vi "Autonomous Independent.vi"   [LabVIEW 2017] (continued)
                        frame #5 {
                          n2054 = global write "Robot Global Data.vi" "Current State"(TRUE ("Current State")) -> ()
                          n2055 = Wait (ms)(milliseconds to wait=u32 300) -> ()  [unwired: 1 out]
                        }
                      }
                    }
                    frame "L" {
                      n2056 = flat-sequence {
                        tunnel: w6977 -> [w6994]
                        tunnel: w6976 -> [w6993]
                        tunnel: [w6996] -> w6991
                        tunnel: [w6995] -> w6990
                        tunnel: w6991 -> [w7003]
                        tunnel: w6990 -> [w7002]
                        tunnel: [w7003] -> w6986
                        tunnel: [w7002] -> w6987
                        tunnel: [w7000] -> w6988
                        tunnel: [w6999] -> w6989
                        tunnel: w6974 -> [w6998]
                        tunnel: w6975 -> [w6997]
                        tunnel: w6989 -> [w7004]
                        tunnel: w6988 -> [w7005]
                        tunnel: w6987 -> [w7008]
                        tunnel: w6986 -> [w7009]
                        tunnel: [w7007] -> w6985
                        tunnel: [w7006] -> w6984
                        tunnel: [w7005] -> w6983
                        tunnel: [w7004] -> w6982
                        tunnel: w6985 -> [w7037]
                        tunnel: [w7037] -> w6981
                        tunnel: w6984 -> [w7036]
                        tunnel: [w7036] -> w6980
                        tunnel: w6983 -> [w7035]
                        tunnel: [w7033] -> w6979
                        tunnel: w6982 -> [w7034]
                        tunnel: [w7032] -> w6978
                        tunnel: w6981 -> [w7047]
                        tunnel: w6980 -> [w7046]
                        tunnel: w6979 -> [w7041]
                        tunnel: w6978 -> [w7039]
                        tunnel: [w7045] -> w6971
                        tunnel: [w7044] -> w6968
                        tunnel: [w7040] -> w6965
                        tunnel: [w7038] -> w6962
                        tunnel: w6961 -> [w7043]
                        tunnel: [w7052] -> w6972
                        tunnel: w6971 -> [w7052]
                        tunnel: [w7051] -> w6969
                        tunnel: w6968 -> [w7051]
                        tunnel: [w7050] -> w6966
                        tunnel: w6965 -> [w7050]
                        tunnel: [w7049] -> w6963
                        tunnel: w6962 -> [w7049]
                        tunnel: [w7065] -> w6973
                        tunnel: w6972 -> [w7065]
                        tunnel: [w7064] -> w6970
                        tunnel: w6969 -> [w7064]
                        tunnel: [w7061] -> w6967
                        tunnel: w6966 -> [w7063]
                        tunnel: [w7060] -> w6964
                        tunnel: w6963 -> [w7062]
                        tunnel: [w7055] -> w6960
                        tunnel: w6973 -> [w7079]
                        tunnel: w6970 -> [w7078]
                        tunnel: w6967 -> [w7077]
                        tunnel: w6964 -> [w7076]
                        tunnel: w6960 -> [w7074]
                        frame #0 {
                          n2057 = call "PID turning.vi"("Angle"=170.0, "GyroDevRef"=w6993, "RobotDriveDevRef"=w6994) -> ("GyroDevRef 2"=w6995:T8, "RobotDriveDevRef 2"=w6996:T1)  [unwired: 7 in]
                        }
                        frame #1 {
                          n2058 = call <vilib>:"WPI_EncoderReset.vi"("EncoderDevRef"=w6998) -> ("EncoderDevRef"=w6999:T11)  [unwired: 9 in, 1 out]
                          n2059 = Wait (ms)(milliseconds to wait=u32 10) -> ()  [unwired: 1 out]
                          n2060 = call <vilib>:"WPI_EncoderReset.vi"("EncoderDevRef"=w6997) -> ("EncoderDevRef"=w7000:T11)  [unwired: 9 in, 1 out]
                        }
                        frame #2 {
                          n2061 = global read "Robot Global Data.vi" "Axes"() -> (w7016:dbl[])
                          n2062 = Wait (ms)(milliseconds to wait=u32 400) -> ()  [unwired: 1 out]
                          n2063 = Array To Cluster(array=w7016) -> (cluster=w7017:T15)
                          n2064 = global read "Robot Global Data.vi" "PIXY Output"() -> (w7010:T16)
                          n2065 = Bundle By Name(cluster=w7017, "Axes[1]"=1.0) -> (w7018:T15)
                          n2066 = Unbundle By Name(w7010) -> ("SIGNATURE NUMBER"=w7013:u16)
                          n2067 = global read "Robot Global Data.vi" "Cube Signature"() -> (w7012:dbl)
                          n2068 = Equal?(x=w7013, y=w7012) -> (x = y?=w7011:bool)
                          n2069 = Cluster To Array(cluster=w7018) -> (array=w7019:dbl[])
                          n2070 = global write "Robot Global Data.vi" "Axes"(w7019) -> ()
                          n2071 = case shown="True" w7011 {
                            tunnel: [w7026 w7029] -> w7006
                            tunnel: [w7027 w7028] -> w7007
                            tunnel: w7009 -> [w7021 w7028]
                            tunnel: w7008 -> [w7020 w7029]
                            frame True {
                              n2072 = call <vilib>:"WPI_GyroGetAngle.vi"("GyroDevRef"=w7020) -> ("Angle"=w7025:dbl, "GyroDevRef"=w7026:T8)  [unwired: 6 in, 3 out]
                              n2073 = In Range and Coerce(upper limit=170.0, x=w7025, lower limit=155.0) -> (coerced(x)=w7024:dbl)  [unwired: 1 out]
                              n2074 = global write "Robot Global Data.vi" "Tracked Angle"(w7024) -> ()
                              n2075 = call "PID vision.vi"("RobotDriveDevRef in"=w7021) -> ("RobotDriveDevRef out"=w7027:T1)  [unwired: 9 in, 1 out]
                            }
                            frame False {
                              n2076 = global write "Robot Global Data.vi" "Tracked Angle"(170.0) -> ()
                            }
                          }
                        }
                        frame #3 {
                          n2077 = call <vilib>:"WPI_EncoderReset.vi"("EncoderDevRef"=w7034) -> ("EncoderDevRef"=w7032:T11)  [unwired: 9 in, 1 out]
                          n2078 = Wait (ms)(milliseconds to wait=u32 10) -> ()  [unwired: 1 out]
                          n2079 = call <vilib>:"WPI_EncoderReset.vi"("EncoderDevRef"=w7035) -> ("EncoderDevRef"=w7033:T11)  [unwired: 9 in, 1 out]
                        }
                        frame #4 {
                          n2080 = global read "Robot Global Data.vi" "Tracked Angle"() -> (w7048:dbl)
                          n2081 = call "PID with Infrared.vi"("RobotDriveDevRef"=w7047, "Angle"=w7048, "Encoder Limit"=60.0, "GyroDevRef"=w7046, "Left Encoder"=w7041, "Right Encoder"=w7039, "DigitalInputDevRef"=w7043) -> ("RobotDriveDevRef 2"=w7045:T1, "GyroDevRef 2"=w7044:T8, "Left Encoder 2"=w7040:T11, "Right Encoder 2"=w7038:T11)  [unwired: 4 in, 1 out]
                        }
                        frame #5 {
                          n2082 = global write "Robot Global Data.vi" "Current State"(TRUE ("Current State")) -> ()
                          n2083 = Wait (ms)(milliseconds to wait=u32 500) -> ()  [unwired: 1 out]
                        }
                        frame #6 {
                          n2084 = global read "Robot Global Data.vi" "Axes"() -> (w7071:dbl[])
                          n2085 = global write "Robot Global Data.vi" "Lift_Position"(2.0) -> ()
                          n2086 = Wait (ms)(milliseconds to wait=u32 400) -> ()  [unwired: 1 out]
                          n2087 = Array To Cluster(array=w7071) -> (cluster=w7070:T15)
                          n2088 = Bundle By Name(cluster=w7070, "Axes[1]"=-1.0) -> (w7069:T15)
                          n2089 = call <vilib>:"WPI_EncoderGet.vi"("EncoderDevRef"=w7063) -> ("Distance"=w7059:dbl, "EncoderDevRef"=w7061:T11)  [unwired: 5 in, 4 out]
                          n2090 = call <vilib>:"WPI_EncoderGet.vi"("EncoderDevRef"=w7062) -> ("Distance"=w7058:dbl, "EncoderDevRef"=w7060:T11)  [unwired: 5 in, 4 out]
                          n2091 = Add(x=w7059, y=w7058) -> (x+y=w7057:dbl)
                          n2092 = Cluster To Array(cluster=w7069) -> (array=w7068:dbl[])
                          n2093 = global write "Robot Global Data.vi" "Axes"(w7068) -> ()
                          n2094 = Divide(x=w7057, y=2.0) -> (x/y=w7055:dbl)
                        }
                        frame #7 {
                          n2095 = Add(x=w7074, y=15.0 ("Distance")) -> (x+y=w7073:dbl)
                          n2096 = global read "Robot Global Data.vi" "Tracked Angle"() -> (w7080:dbl)
                          n2097 = call "PID Distance.vi"("Distance"=w7073, "Angle"=w7080, "RightEncoder"=w7076, "LeftEncoder"=w7077, "GyroDevRef"=w7078, "RobotDriveDevRef"=w7079) -> ()  [unwired: 2 in, 4 out]
                        }
                        frame #8 {
                          n2098 = global read "Robot Global Data.vi" "Axes"() -> (w7086:dbl[])
                          n2099 = Wait (ms)(milliseconds to wait=u32 200) -> ()  [unwired: 1 out]
                          n2100 = Array To Cluster(array=w7086) -> (cluster=w7085:T15)
                          n2101 = Bundle By Name(cluster=w7085, "Axes[1]"=0.5) -> (w7084:T15)
                          n2102 = Cluster To Array(cluster=w7084) -> (array=w7083:dbl[])
                          n2103 = global write "Robot Global Data.vi" "Axes"(w7083) -> ()
                        }
                        frame #9 {
                          n2104 = global write "Robot Global Data.vi" "Current State"(FALSE ("Current State")) -> ()
                        }
                      }
                    }
                    frame Default {
                    }
                  }
                }
              }
            }
            frame "R" {
              n2105 = flat-sequence {
                tunnel: [w7154] -> w7142
                tunnel: [w7153] -> w7143
                tunnel: [w7151] -> w7144
                tunnel: [w7152] -> w7145
                tunnel: w7101 -> [w7150]
                tunnel: w7100 -> [w7149]
                tunnel: w7099 -> [w7148]
                tunnel: w7098 -> [w7147]
                tunnel: [w7174] -> w7141
                tunnel: w7145 -> [w7170]
                tunnel: w7144 -> [w7171]
                tunnel: w7143 -> [w7173]
                tunnel: w7142 -> [w7175]
                tunnel: [w7172] -> w7140
                tunnel: [w7171] -> w7139
                tunnel: [w7170] -> w7138
                tunnel: w7141 -> [w7185]
                tunnel: [w7185] -> w7137
                tunnel: w7140 -> [w7184]
                tunnel: [w7184] -> w7136
                tunnel: [w7183] -> w7135
                tunnel: [w7182] -> w7134
                tunnel: w7139 -> [w7180]
                tunnel: w7138 -> [w7179]
                tunnel: w7137 -> [w7191]
                tunnel: [w7189] -> w7133
                tunnel: w7136 -> [w7190]
                tunnel: [w7188] -> w7132
                tunnel: w7135 -> [w7193]
                tunnel: w7134 -> [w7192]
                tunnel: [w7187] -> w7131
                tunnel: [w7186] -> w7130
                tunnel: w7133 -> [w7200]
                tunnel: [w7199] -> w7129
                tunnel: [w7198] -> w7128
                tunnel: w7132 -> [w7198]
                tunnel: [w7197] -> w7127
                tunnel: w7131 -> [w7197]
                tunnel: [w7196] -> w7126
                tunnel: w7130 -> [w7196]
                tunnel: [w7211] -> w7125
                tunnel: w7129 -> [w7211]
                tunnel: [w7210] -> w7124
                tunnel: w7128 -> [w7210]
                tunnel: [w7209] -> w7123
                tunnel: w7127 -> [w7209]
                tunnel: [w7208] -> w7122
                tunnel: w7126 -> [w7208]
                tunnel: w7125 -> [w7216]
                tunnel: w7124 -> [w7217]
                tunnel: [w7217] -> w7121
                tunnel: [w7216] -> w7120
                tunnel: [w7215] -> w7119
                tunnel: w7123 -> [w7215]
                tunnel: [w7214] -> w7118
                tunnel: w7122 -> [w7214]
                tunnel: [w7230] -> w7117
                tunnel: w7121 -> [w7232]
                tunnel: w7120 -> [w7231]
                tunnel: w7119 -> [w7227]
                tunnel: w7118 -> [w7226]
                tunnel: [w7225] -> w7116
                tunnel: [w7224] -> w7115
                tunnel: [w7223] -> w7114
                tunnel: w7117 -> [w7239]
                tunnel: w7116 -> [w7238]
                tunnel: [w7237] -> w7096
                tunnel: w7115 -> [w7237]
                tunnel: [w7236] -> w7094
                tunnel: w7114 -> [w7236]
                tunnel: [w7235] -> w7092
                tunnel: [w7234] -> w7090
                tunnel: w7096 -> [w7248]
                tunnel: [w7245] -> w7095
                tunnel: w7094 -> [w7247]
                tunnel: [w7244] -> w7093
                tunnel: w7092 -> [w7249]
                tunnel: [w7246] -> w7091
                tunnel: w7090 -> [w7243]
                tunnel: [w7242] -> w7088
                tunnel: w7095 -> [w7274]
                tunnel: w7093 -> [w7273]
                tunnel: [w7271] -> w7113
                tunnel: w7091 -> [w7271]
                tunnel: [w7268] -> w7112
                tunnel: [w7270] -> w7111
                tunnel: [w7269] -> w7110
                tunnel: w7088 -> [w7268]
                tunnel: w7113 -> [w7284]
                tunnel: w7112 -> [w7282]
                tunnel: w7111 -> [w7278]
                tunnel: w7110 -> [w7276]
                tunnel: [w7283] -> w7109
                tunnel: [w7281] -> w7108
                tunnel: [w7277] -> w7107
                tunnel: [w7275] -> w7106
                tunnel: w7089 -> [w7280]
                tunnel: [w7295] -> w7105
                tunnel: [w7292] -> w7104
                tunnel: [w7294] -> w7103
                tunnel: [w7293] -> w7102
                tunnel: w7106 -> [w7292]
                tunnel: w7107 -> [w7293]
                tunnel: w7108 -> [w7294]
                tunnel: w7109 -> [w7295]
                tunnel: w7105 -> [w7302]
                tunnel: w7104 -> [w7301]
                tunnel: w7103 -> [w7300]
                tunnel: w7102 -> [w7299]
                tunnel: w7097 -> [w7298]
                frame #0 {
                  n2106 = while {
                    tunnel: [w7159] -> w7146
                    stop <- w7158 stop-if-true
                    w7162 = 100.0 ("y")
                    w7165 = 20.0 ("y")
                    n2107 = global read "Robot Global Data.vi" "Distance 2"() -> (w7160:dbl)
                    n2108 = global read "Robot Global Data.vi" "Distance"() -> (w7161:dbl)
                    n2109 = Greater?(x=w7161, y=w7165) -> (0:w7167:bool)
                    n2110 = Greater?(x=w7160, y=w7165) -> (0:w7166:bool)
                    n2111 = Greater?(x=w7161, y=w7162) -> (0:w7164:bool)
                    n2112 = Greater?(x=w7160, y=w7162) -> (0:w7163:bool)
                    n2113 = Or(x=w7167, y=w7166) -> (x .or. y?=w7157:bool)
                    n2114 = Or(x=w7164, y=w7163) -> (x .or. y?=w7158:bool)
                    n2115 = global write "Robot Global Data.vi" "Raise_Mast"(w7157) -> ()
                    n2116 = case shown="True" w7158 {
                      tunnel: [0.0 2.0] -> w7159
                      frame False {
                      }
                      frame True {
                      }
                    }
                  }
                  n2117 = call "PID Distance.vi"("Distance"=295.0, "Angle"=2.0, "RightEncoder"=w7147, "LeftEncoder"=w7148, "GyroDevRef"=w7149, "RobotDriveDevRef"=w7150) -> ("RightEncoder 2"=w7151:T11, "LeftEncoder 2"=w7152:T11, "GyroDevRef 2"=w7153:T8, "RobotDriveDevRef 2"=w7154:T1)  [unwired: 2 in]
                  n2118 = global write "Robot Global Data.vi" "Lift_Position"(w7146) -> ()
                }
                frame #1 {
                  n2119 = call "PID turning.vi"("Angle"=-90.0, "GyroDevRef"=w7173, "RobotDriveDevRef"=w7175) -> ("GyroDevRef 2"=w7172:T8, "RobotDriveDevRef 2"=w7174:T1)  [unwired: 7 in]
                  n2120 = global write "Robot Global Data.vi" "Lift_Position"(3.0) -> ()
                  n2121 = global write "Robot Global Data.vi" "Raise_Mast"(TRUE ("Current State")) -> ()
                }
                frame #2 {
                  n2122 = call <vilib>:"WPI_EncoderReset.vi"("EncoderDevRef"=w7179) -> ("EncoderDevRef"=w7182:T11)  [unwired: 9 in, 1 out]
                  n2123 = Wait (ms)(milliseconds to wait=u32 100) -> ()  [unwired: 1 out]
                  n2124 = call <vilib>:"WPI_EncoderReset.vi"("EncoderDevRef"=w7180) -> ("EncoderDevRef"=w7183:T11)  [unwired: 9 in, 1 out]
                }
                frame #3 {
                  n2125 = call "PID Distance.vi"("Distance"=25.0, "Angle"=-90.0, "RightEncoder"=w7193, "LeftEncoder"=w7192, "GyroDevRef"=w7190, "RobotDriveDevRef"=w7191) -> ("RightEncoder 2"=w7186:T11, "LeftEncoder 2"=w7187:T11, "GyroDevRef 2"=w7188:T8, "RobotDriveDevRef 2"=w7189:T1)  [unwired: 2 in]
                }
                frame #4 {
                  w7201 = 0.0 ("Left axis value")
                  n2126 = global read "Robot Global Data.vi" "Axes"() -> (w7204:dbl[])
                  n2127 = Wait (ms)(milliseconds to wait=u32 500) -> ()  [unwired: 1 out]
                  n2128 = Array To Cluster(array=w7204) -> (cluster=w7203:T15)
                  n2129 = Bundle By Name(cluster=w7203, "Axes[1]"=0.25) -> (w7206:T15)
                  n2130 = Cluster To Array(cluster=w7206) -> (array=w7205:dbl[])
                  n2131 = call <vilib>:"WPI_RobotDriveTankDrive.vi"("Right axis value"=w7201, "Left axis value"=w7201, "RobotDriveDevRef"=w7200) -> ("RobotDriveDevRef"=w7199:T1)  [unwired: 6 in, 2 out]
                  n2132 = global write "Robot Global Data.vi" "Axes"(w7205) -> ()
                }
                frame #5 {
                  n2133 = global write "Robot Global Data.vi" "Current State"(FALSE ("Current State")) -> ()
                  n2134 = Wait (ms)(milliseconds to wait=u32 400) -> ()  [unwired: 1 out]
                }
                frame #6 {
                  n2135 = global read "Robot Global Data.vi" "Axes"() -> (w7219:dbl[])
                  n2136 = Array To Cluster(array=w7219) -> (cluster=w7218:T15)
                  n2137 = Bundle By Name(cluster=w7218, "Axes[1]"=-1.0) -> (w7221:T15)
                  n2138 = Cluster To Array(cluster=w7221) -> (array=w7220:dbl[])
                  n2139 = global write "Robot Global Data.vi" "Axes"(w7220) -> ()
                }
                frame #7 {
                  # "7 for A bot"
                  n2140 = call "PID Distance.vi"("Distance"=7.0, "Angle"=-90.0, "RightEncoder"=w7226, "LeftEncoder"=w7227, "GyroDevRef"=w7232, "RobotDriveDevRef"=w7231) -> ("RightEncoder 2"=w7223:T11, "LeftEncoder 2"=w7224:T11, "GyroDevRef 2"=w7225:T8, "RobotDriveDevRef 2"=w7230:T1)  [unwired: 2 in]
                }
                frame #8 {
                  n2141 = global write "Robot Global Data.vi" "Lift_Position"(1.0) -> ()
                  n2142 = call "PID turning.vi"("Angle"=-170.0, "GyroDevRef"=w7238, "RobotDriveDevRef"=w7239) -> ("GyroDevRef 2"=w7234:T8, "RobotDriveDevRef 2"=w7235:T1)  [unwired: 7 in]
                }
                frame #9 {
                  n2143 = global read "Robot Global Data.vi" "PIXY Output"() -> (w7252:T16)
                  n2144 = Unbundle By Name(w7252) -> ("SIGNATURE NUMBER"=w7251:u16)
                  n2145 = global read "Robot Global Data.vi" "Cube Signature"() -> (w7241:dbl)
                  n2146 = Equal?(x=w7251, y=w7241) -> (x = y?=w7250:bool)
                  n2147 = case shown="True" w7250 {
                    tunnel: [w7260 w7264] -> w7244
                    tunnel: [w7259 w7265] -> w7245
                    tunnel: [w7261 w7266] -> w7246
                    tunnel: w7248 -> [w7259 w7265]
                    tunnel: w7247 -> [w7260 w7264]
                    tunnel: w7249 -> [w7262 w7266]
                    tunnel: w7243 -> [w7254 w7263]
                    tunnel: [w7253 w7263] -> w7242
                    frame True {
                      # "-150_-170"
                      n2148 = call <vilib>:"WPI_GyroGetAngle.vi"("GyroDevRef"=w7254) -> ("Angle"=w7257:dbl, "GyroDevRef"=w7253:T8)  [unwired: 6 in, 3 out]
                      n2149 = In Range and Coerce(upper limit=-150.0, x=w7257, lower limit=-170.0) -> (coerced(x)=w7258:dbl)  [unwired: 1 out]
                      n2150 = global write "Robot Global Data.vi" "Tracked Angle"(w7258) -> ()
                      n2151 = call "PID vision.vi"("RobotDriveDevRef in"=w7262) -> ("RobotDriveDevRef out"=w7261:T1)  [unwired: 9 in, 1 out]
                    }
                    frame False {
                      n2152 = global write "Robot Global Data.vi" "Tracked Angle"(-165.0) -> ()
                    }
                  }
                }
                frame #10 {
                  n2153 = call <vilib>:"WPI_EncoderReset.vi"("EncoderDevRef"=w7274) -> ("EncoderDevRef"=w7270:T11)  [unwired: 9 in, 1 out]
                  n2154 = Wait (ms)(milliseconds to wait=u32 10) -> ()  [unwired: 1 out]
                  n2155 = call <vilib>:"WPI_EncoderReset.vi"("EncoderDevRef"=w7273) -> ("EncoderDevRef"=w7269:T11)  [unwired: 9 in, 1 out]
                }
                frame #11 {
                  n2156 = global write "Robot Global Data.vi" "Lift_Position"(0.0) -> ()
                  n2157 = global read "Robot Global Data.vi" "Axes"() -> (w7289:dbl[])
                  n2158 = Array To Cluster(array=w7289) -> (cluster=w7288:T15)
                  n2159 = global read "Robot Global Data.vi" "Tracked Angle"() -> (w7285:dbl)
                  n2160 = Bundle By Name(cluster=w7288, "Axes[1]"=1.0) -> (w7291:T15)
                  n2161 = call "PID with Infrared.vi"("RobotDriveDevRef"=w7284, "Angle"=w7285, "Encoder Limit"=120.0, "GyroDevRef"=w7282, "Left Encoder"=w7278, "Right Encoder"=w7276, "DigitalInputDevRef"=w7280) -> ("RobotDriveDevRef 2"=w7283:T1, "GyroDevRef 2"=w7281:T8, "Left Encoder 2"=w7277:T11, "Right Encoder 2"=w7275:T11)  [unwired: 4 in, 1 out]
                  n2162 = Cluster To Array(cluster=w7291) -> (array=w7290:dbl[])
                  n2163 = global write "Robot Global Data.vi" "Axes"(w7290) -> ()
                }
                frame #12 {
                  n2164 = global write "Robot Global Data.vi" "Current State"(TRUE ("Current State")) -> ()
                  n2165 = Wait (ms)(milliseconds to wait=u32 750) -> ()  [unwired: 1 out]
                }
                frame #13 {
                  n2166 = case shown="\"L\"" w7298 {
                    tunnel: w7302 -> [w7309 w7373 _]
                    tunnel: w7301 -> [w7306 w7372 _]
                    tunnel: w7300 -> [w7308 w7371 _]
                    tunnel: w7299 -> [w7307 w7370 _]
                    frame "R" {
                      n2167 = flat-sequence {
                        tunnel: w7307 -> [w7318]
                        tunnel: w7306 -> [w7317]
                        tunnel: [w7316] -> w7305
                        tunnel: [w7315] -> w7304
                        tunnel: [w7310] -> w7303
                        tunnel: w7309 -> [w7333]
                        tunnel: w7308 -> [w7332]
                        tunnel: w7305 -> [w7330]
                        tunnel: w7304 -> [w7329]
                        tunnel: w7303 -> [w7326]
                        frame #0 {
                          n2168 = global read "Robot Global Data.vi" "Axes"() -> (w7323:dbl[])
                          n2169 = global write "Robot Global Data.vi" "Lift_Position"(2.0) -> ()
                          n2170 = Wait (ms)(milliseconds to wait=u32 250) -> ()  [unwired: 1 out]
                          n2171 = Array To Cluster(array=w7323) -> (cluster=w7322:T15)
                          n2172 = Bundle By Name(cluster=w7322, "Axes[1]"=-1.0) -> (w7325:T15)
                          n2173 = call <vilib>:"WPI_EncoderGet.vi"("EncoderDevRef"=w7318) -> ("Distance"=w7314:dbl, "EncoderDevRef"=w7316:T11)  [unwired: 5 in, 4 out]
                          n2174 = call <vilib>:"WPI_EncoderGet.vi"("EncoderDevRef"=w7317) -> ("Distance"=w7313:dbl, "EncoderDevRef"=w7315:T11)  [unwired: 5 in, 4 out]
                          n2175 = Add(x=w7314, y=w7313) -> (x+y=w7312:dbl)
                          n2176 = Cluster To Array(cluster=w7325) -> (array=w7324:dbl[])
                          n2177 = global write "Robot Global Data.vi" "Axes"(w7324) -> ()
                          n2178 = Divide(x=w7312, y=2.0) -> (x/y=w7310:dbl)
                        }
                        frame #1 {
                          n2179 = Add(x=w7326, y=15.0 ("Distance")) -> (x+y=w7327:dbl)
                          n2180 = global read "Robot Global Data.vi" "Tracked Angle"() -> (w7331:dbl)
                          n2181 = call "PID Distance.vi"("Distance"=w7327, "Angle"=w7331, "RightEncoder"=w7329, "LeftEncoder"=w7330, "GyroDevRef"=w7332, "RobotDriveDevRef"=w7333) -> ()  [unwired: 2 in, 4 out]
                        }
                        frame #2 {
                          n2182 = global read "Robot Global Data.vi" "Axes"() -> (w7337:dbl[])
                          n2183 = Wait (ms)(milliseconds to wait=u32 200) -> ()  [unwired: 1 out]
                          n2184 = Array To Cluster(array=w7337) -> (cluster=w7336:T15)
                          n2185 = Bundle By Name(cluster=w7336, "Axes[1]"=0.5) -> (w7339:T15)
                          n2186 = Cluster To Array(cluster=w7339) -> (array=w7338:dbl[])
                          n2187 = global write "Robot Global Data.vi" "Axes"(w7338) -> ()
                        }
                        frame #3 {
                          n2188 = global write "Robot Global Data.vi" "Current State"(FALSE ("Current State")) -> ()
                          n2189 = Wait (ms)(milliseconds to wait=u32 500) -> ()  [unwired: 1 out]
                        }
                      }
                    }
                    frame "L" {
                      n2190 = flat-sequence {
                        tunnel: w7373 -> [w7384]
                        tunnel: w7372 -> [w7389]
                        tunnel: w7371 -> [w7383]
                        tunnel: w7370 -> [w7382]
                        tunnel: [w7388] -> w7369
                        tunnel: [w7387] -> w7368
                        tunnel: [w7386] -> w7366
                        tunnel: [w7385] -> w7364
                        tunnel: w7369 -> [w7397]
                        tunnel: w7368 -> [w7396]
                        tunnel: [w7395] -> w7367
                        tunnel: w7366 -> [w7395]
                        tunnel: [w7394] -> w7365
                        tunnel: w7364 -> [w7394]
                        tunnel: [w7393] -> w7362
                        tunnel: [w7392] -> w7360
                        tunnel: w7367 -> [w7404]
                        tunnel: w7365 -> [w7403]
                        tunnel: [w7402] -> w7363
                        tunnel: w7362 -> [w7402]
                        tunnel: [w7401] -> w7361
                        tunnel: w7360 -> [w7401]
                        tunnel: [w7400] -> w7359
                        tunnel: [w7399] -> w7358
                        tunnel: w7363 -> [w7414]
                        tunnel: w7361 -> [w7413]
                        tunnel: w7359 -> [w7412]
                        tunnel: w7358 -> [w7411]
                        tunnel: [w7410] -> w7357
                        tunnel: [w7409] -> w7356
                        tunnel: [w7407] -> w7355
                        tunnel: [w7406] -> w7354
                        tunnel: [w7420] -> w7353
                        tunnel: [w7419] -> w7352
                        tunnel: [w7418] -> w7351
                        tunnel: [w7417] -> w7350
                        tunnel: w7354 -> [w7417]
                        tunnel: w7355 -> [w7418]
                        tunnel: w7356 -> [w7419]
                        tunnel: w7357 -> [w7420]
                        tunnel: [w7430] -> w7343
                        tunnel: w7353 -> [w7430]
                        tunnel: [w7429] -> w7345
                        tunnel: w7352 -> [w7429]
                        tunnel: [w7428] -> w7347
                        tunnel: w7351 -> [w7428]
                        tunnel: [w7427] -> w7349
                        tunnel: w7350 -> [w7427]
                        tunnel: w7349 -> [w7442]
                        tunnel: [w7442] -> w7348
                        tunnel: w7347 -> [w7441]
                        tunnel: [w7441] -> w7346
                        tunnel: w7345 -> [w7440]
                        tunnel: [w7440] -> w7344
                        tunnel: w7343 -> [w7439]
                        tunnel: [w7439] -> w7342
                        tunnel: w7348 -> [w7443]
                        tunnel: w7346 -> [w7444]
                        tunnel: w7344 -> [w7445]
                        tunnel: w7342 -> [w7446]
                        frame #0 {
                          n2191 = global read "Robot Global Data.vi" "Axes"() -> (w7378:dbl[])
                          n2192 = global write "Robot Global Data.vi" "Lift_Position"(2.0) -> ()
                          n2193 = Wait (ms)(milliseconds to wait=u32 250) -> ()  [unwired: 1 out]
                          n2194 = Array To Cluster(array=w7378) -> (cluster=w7377:T15)
                          n2195 = Bundle By Name(cluster=w7377, "Axes[1]"=-1.0) -> (w7380:T15)
                          n2196 = Cluster To Array(cluster=w7380) -> (array=w7379:dbl[])
                          n2197 = global write "Robot Global Data.vi" "Axes"(w7379) -> ()
                        }
                        frame #1 {
                          n2198 = global read "Robot Global Data.vi" "Tracked Angle"() -> (w7381:dbl)
                          n2199 = call "PID Distance.vi"("Distance"=-10.0, "Angle"=w7381, "RightEncoder"=w7389, "LeftEncoder"=w7382, "GyroDevRef"=w7383, "RobotDriveDevRef"=w7384) -> ("RightEncoder 2"=w7385:T11, "LeftEncoder 2"=w7386:T11, "GyroDevRef 2"=w7387:T8, "RobotDriveDevRef 2"=w7388:T1)  [unwired: 2 in]
                        }
                        frame #2 {
                          n2200 = call "PID turning.vi"("Angle"=-90.0, "GyroDevRef"=w7396, "RobotDriveDevRef"=w7397) -> ("GyroDevRef 2"=w7392:T8, "RobotDriveDevRef 2"=w7393:T1)  [unwired: 7 in]
                          n2201 = global write "Robot Global Data.vi" "Lift_Position"(3.0) -> ()
                        }
                        frame #3 {
                          n2202 = call <vilib>:"WPI_EncoderReset.vi"("EncoderDevRef"=w7404) -> ("EncoderDevRef"=w7400:T11)  [unwired: 9 in, 1 out]
                          n2203 = Wait (ms)(milliseconds to wait=u32 10) -> ()  [unwired: 1 out]
                          n2204 = call <vilib>:"WPI_EncoderReset.vi"("EncoderDevRef"=w7403) -> ("EncoderDevRef"=w7399:T11)  [unwired: 9 in, 1 out]
                        }
                        frame #4 {
                          n2205 = global write "Robot Global Data.vi" "Lift_Position"(3.0) -> ()
                          n2206 = call "PID Distance.vi"("Distance"=30.0, "Angle"=-90.0, "RightEncoder"=w7411, "LeftEncoder"=w7412, "GyroDevRef"=w7413, "RobotDriveDevRef"=w7414) -> ("RightEncoder 2"=w7406:T11, "LeftEncoder 2"=w7407:T11, "GyroDevRef 2"=w7409:T8, "RobotDriveDevRef 2"=w7410:T1)  [unwired: 2 in]
                        }
                        frame #5 {
                          n2207 = global read "Robot Global Data.vi" "Axes"() -> (w7424:dbl[])
                          n2208 = Wait (ms)(milliseconds to wait=u32 500) -> ()  [unwired: 1 out]
                          n2209 = Array To Cluster(array=w7424) -> (cluster=w7423:T15)
                          n2210 = Bundle By Name(cluster=w7423, "Axes[1]"=0.3) -> (w7426:T15)
                          n2211 = Cluster To Array(cluster=w7426) -> (array=w7425:dbl[])
                          n2212 = global write "Robot Global Data.vi" "Axes"(w7425) -> ()
                        }
                        frame #6 {
                          n2213 = global write "Robot Global Data.vi" "Current State"(FALSE ("Current State")) -> ()
                          n2214 = Wait (ms)(milliseconds to wait=u32 400) -> ()  [unwired: 1 out]
                        }
                        frame #7 {
                          n2215 = global read "Robot Global Data.vi" "Axes"() -> (w7436:dbl[])
                          n2216 = Wait (ms)(milliseconds to wait=u32 250) -> ()  [unwired: 1 out]
                          n2217 = Array To Cluster(array=w7436) -> (cluster=w7435:T15)
                          n2218 = Bundle By Name(cluster=w7435, "Axes[1]"=-1.0) -> (w7438:T15)
                          n2219 = Cluster To Array(cluster=w7438) -> (array=w7437:dbl[])
                          n2220 = global write "Robot Global Data.vi" "Axes"(w7437) -> ()
                        }
                        frame #8 {
                          n2221 = call "PID Distance.vi"("Distance"=10.0, "Angle"=-90.0, "RightEncoder"=w7443, "LeftEncoder"=w7444, "GyroDevRef"=w7445, "RobotDriveDevRef"=w7446) -> ()  [unwired: 2 in, 4 out]
                        }
                        frame #9 {
                          n2222 = global write "Robot Global Data.vi" "Lift_Position"(1.0) -> ()
                        }
                      }
                    }
                    frame Default {
                    }
                  }
                }
              }
            }
            frame Default {
              n2223 = flat-sequence {
                tunnel: w7451 -> [w7459]
                tunnel: w7450 -> [w7458]
                tunnel: w7452 -> [w7456]
                tunnel: [w7457] -> w7454
                tunnel: w7453 -> [w7455]
                tunnel: w7454 -> [w7462]
                frame #0 {
                  n2224 = call "PID Distance.vi"("Distance"=90.0, "Angle"=0.0, "RightEncoder"=w7455, "LeftEncoder"=w7456, "GyroDevRef"=w7458, "RobotDriveDevRef"=w7459) -> ("RobotDriveDevRef 2"=w7457:T1)  [unwired: 2 in, 3 out]
                }
                frame #1 {
                  w7463 = 0.0
                  n2225 = call <vilib>:"WPI_RobotDriveTankDrive.vi"("Right axis value"=w7463, "Left axis value"=w7463, "RobotDriveDevRef"=w7462) -> ()  [unwired: 6 in, 3 out]
                }
              }
            }
          }
        }
      }
    }
    frame "Right Switch" {
      n2226 = flat-sequence {
        tunnel: w7473 -> [w7498]
        tunnel: w7472 -> [w7496]
        tunnel: w7471 -> [w7495]
        tunnel: w7470 -> [w7494]
        tunnel: [w7493] -> w7468
        tunnel: [w7492] -> w7467
        tunnel: [w7491] -> w7466
        tunnel: [w7490] -> w7465
        tunnel: w7464 -> [w7483]
        tunnel: w7469 -> [w7503]
        tunnel: w7468 -> [w7502]
        tunnel: w7467 -> [w7501]
        tunnel: w7466 -> [w7500]
        tunnel: w7465 -> [w7499]
        frame #0 {
          w7497 = 0.0 ("Left axis value")
          n2227 = global read "Robot Global Data.vi" "Axes"() -> (w7476:dbl[])
          n2228 = Multiply(x=w7483, y=1000.0) -> (x*y=w7484:dbl)
          n2229 = global write "Robot Global Data.vi" "Lift_Position"(0.0) -> ()
          n2230 = global write "Robot Global Data.vi" "Raise_Mast"(FALSE ("Current State")) -> ()
          n2231 = global write "Robot Global Data.vi" "Current State"(TRUE ("Current State")) -> ()
          n2232 = Wait (ms)(milliseconds to wait=10) -> ()  [unwired: 1 out]
          n2233 = Array To Cluster(array=w7476) -> (cluster=w7475:T15)
          n2234 = Bundle By Name(cluster=w7475, "Axes[1]"=-1.0) -> (w7478:T15)
          n2235 = Greater?(x=w7484, y=11000.0) -> (0:w7486:bool)
          n2236 = Equal?(x=w7484, y=0.0) -> (x = y?=w7487:bool)
          n2237 = Or(x=w7486, y=w7487) -> ()  [unwired: 1 out]
          n2238 = Cluster To Array(cluster=w7478) -> (array=w7477:dbl[])
          n2239 = call <vilib>:"WPI_GyroReset.vi"("GyroDevRef"=w7494) -> ("GyroDevRef"=w7490:T8)  [unwired: 9 in, 1 out]
          n2240 = call <vilib>:"WPI_EncoderReset.vi"("EncoderDevRef"=w7496) -> ("EncoderDevRef"=w7492:T11)  [unwired: 9 in, 1 out]
          n2241 = global write "Robot Global Data.vi" "Axes"(w7477) -> ()
          n2242 = call <vilib>:"WPI_EncoderReset.vi"("EncoderDevRef"=w7495) -> ("EncoderDevRef"=w7491:T11)  [unwired: 9 in, 1 out]
          n2243 = call <vilib>:"WPI_RobotDriveTankDrive.vi"("Right axis value"=w7497, "Left axis value"=w7497, "RobotDriveDevRef"=w7498) -> ("RobotDriveDevRef"=w7493:T1)  [unwired: 6 in, 2 out]
        }
        frame #1 {
          n2244 = case shown="\"R\"" w7503 {
            tunnel: w7502 -> [w7524 w7605 w7714]
            tunnel: w7501 -> [w7523 w7602 w7711]
            tunnel: w7500 -> [w7522 w7603 w7712]
            tunnel: w7499 -> [w7521 w7604 w7713]
            frame "R" {
              n2245 = flat-sequence {
                tunnel: w7521 -> [w7529]
                tunnel: w7522 -> [w7531]
                tunnel: w7523 -> [w7533]
                tunnel: w7524 -> [w7527]
                tunnel: [w7526] -> w7507
                tunnel: [w7532] -> w7506
                tunnel: [w7530] -> w7505
                tunnel: [w7528] -> w7504
                tunnel: [w7538] -> w7520
                tunnel: [w7537] -> w7519
                tunnel: [w7536] -> w7517
                tunnel: [w7535] -> w7516
                tunnel: w7507 -> [w7542]
                tunnel: w7506 -> [w7540]
                tunnel: w7505 -> [w7541]
                tunnel: w7504 -> [w7543]
                tunnel: w7520 -> [w7551]
                tunnel: w7519 -> [w7550]
                tunnel: [w7549] -> w7515
                tunnel: [w7548] -> w7513
                tunnel: [w7547] -> w7511
                tunnel: w7517 -> [w7547]
                tunnel: [w7546] -> w7509
                tunnel: w7516 -> [w7546]
                tunnel: w7515 -> [w7562]
                tunnel: [w7561] -> w7514
                tunnel: w7513 -> [w7567]
                tunnel: [w7567] -> w7512
                tunnel: w7511 -> [w7566]
                tunnel: [w7564] -> w7510
                tunnel: w7509 -> [w7565]
                tunnel: [w7563] -> w7508
                tunnel: w7514 -> [w7572]
                tunnel: [w7571] -> w7518
                tunnel: w7512 -> [w7570]
                tunnel: w7510 -> [w7569]
                tunnel: w7508 -> [w7568]
                tunnel: w7518 -> [w7582]
                frame #0 {
                  n2246 = call "PID Distance.vi"("Distance"=20.0, "Angle"=0.0, "RightEncoder"=w7533, "LeftEncoder"=w7531, "GyroDevRef"=w7529, "RobotDriveDevRef"=w7527) -> ("RightEncoder 2"=w7532:T11, "LeftEncoder 2"=w7530:T11, "GyroDevRef 2"=w7528:T8, "RobotDriveDevRef 2"=w7526:T1)  [unwired: 2 in]
                }
                frame #1 {
                  n2247 = call "PID Distance.vi"("Distance"=120.0, "Angle"=0.0, "RightEncoder"=w7540, "LeftEncoder"=w7541, "GyroDevRef"=w7543, "RobotDriveDevRef"=w7542) -> ("RightEncoder 2"=w7535:T11, "LeftEncoder 2"=w7536:T11, "GyroDevRef 2"=w7537:T8, "RobotDriveDevRef 2"=w7538:T1)  [unwired: 2 in]
                  n2248 = global write "Robot Global Data.vi" "Raise_Mast"(TRUE ("Current State")) -> ()
                }
                frame #2 {
                  n2249 = global read "Robot Global Data.vi" "Axes"() -> (w7554:dbl[])
                  n2250 = global write "Robot Global Data.vi" "Lift_Position"(2.0) -> ()
                  n2251 = call "PID turning.vi"("Angle"=-90.0, "GyroDevRef"=w7550, "RobotDriveDevRef"=w7551) -> ("GyroDevRef 2"=w7548:T8, "RobotDriveDevRef 2"=w7549:T1)  [unwired: 7 in]
                  n2252 = Array To Cluster(array=w7554) -> (cluster=w7553:T15)
                  n2253 = Bundle By Name(cluster=w7553, "Axes[1]"=1.0) -> (w7556:T15)
                  n2254 = Cluster To Array(cluster=w7556) -> (array=w7555:dbl[])
                  n2255 = global write "Robot Global Data.vi" "Axes"(w7555) -> ()
                }
                frame #3 {
                  w7560 = 0.0 ("Left axis value")
                  n2256 = call <vilib>:"WPI_EncoderReset.vi"("EncoderDevRef"=w7566) -> ("EncoderDevRef"=w7564:T11)  [unwired: 9 in, 1 out]
                  n2257 = call <vilib>:"WPI_RobotDriveTankDrive.vi"("Right axis value"=w7560, "Left axis value"=w7560, "RobotDriveDevRef"=w7562) -> ("RobotDriveDevRef"=w7561:T1)  [unwired: 6 in, 2 out]
                  n2258 = Wait (ms)(milliseconds to wait=u32 10) -> ()  [unwired: 1 out]
                  n2259 = call <vilib>:"WPI_EncoderReset.vi"("EncoderDevRef"=w7565) -> ("EncoderDevRef"=w7563:T11)  [unwired: 9 in, 1 out]
                }
                frame #4 {
                  n2260 = call "PID Distance.vi"("Distance"=20.0, "Angle"=-90.0, "RightEncoder"=w7568, "LeftEncoder"=w7569, "GyroDevRef"=w7570, "RobotDriveDevRef"=w7572) -> ("RobotDriveDevRef 2"=w7571:T1)  [unwired: 2 in, 3 out]
                }
                frame #5 {
                  w7581 = 0.0 ("Left axis value")
                  n2261 = global read "Robot Global Data.vi" "Axes"() -> (w7577:dbl[])
                  n2262 = call <vilib>:"WPI_RobotDriveTankDrive.vi"("Right axis value"=w7581, "Left axis value"=w7581, "RobotDriveDevRef"=w7582) -> ()  [unwired: 6 in, 3 out]
                  n2263 = global write "Robot Global Data.vi" "Current State"(FALSE ("Current State")) -> ()
                  n2264 = Array To Cluster(array=w7577) -> (cluster=w7576:T15)
                  n2265 = Bundle By Name(cluster=w7576, "Axes[1]"=0.0) -> (w7579:T15)
                  n2266 = Cluster To Array(cluster=w7579) -> (array=w7578:dbl[])
                  n2267 = global write "Robot Global Data.vi" "Axes"(w7578) -> ()
                }
              }
            }
            frame "L" {
              n2268 = flat-sequence {
                tunnel: w7604 -> [w7626]
                tunnel: w7603 -> [w7625]
                tunnel: w7602 -> [w7624]
                tunnel: w7605 -> [w7627]
                tunnel: [w7623] -> w7601
                tunnel: [w7620] -> w7600
                tunnel: [w7621] -> w7599
                tunnel: [w7622] -> w7598
                tunnel: [w7632] -> w7619
                tunnel: [w7633] -> w7618
                tunnel: [w7630] -> w7617
                tunnel: [w7631] -> w7616
                tunnel: w7601 -> [w7636]
                tunnel: w7600 -> [w7634]
                tunnel: w7599 -> [w7635]
                tunnel: w7598 -> [w7637]
                tunnel: w7619 -> [w7644]
                tunnel: w7618 -> [w7643]
                tunnel: [w7647] -> w7615
                tunnel: w7617 -> [w7647]
                tunnel: [w7646] -> w7614
                tunnel: w7616 -> [w7646]
                tunnel: [w7642] -> w7613
                tunnel: [w7641] -> w7612
                tunnel: w7615 -> [w7654]
                tunnel: w7614 -> [w7653]
                tunnel: [w7652] -> w7611
                tunnel: [w7651] -> w7610
                tunnel: [w7650] -> w7609
                tunnel: w7613 -> [w7650]
                tunnel: [w7648] -> w7608
                tunnel: w7612 -> [w7648]
                tunnel: w7611 -> [w7658]
                tunnel: w7610 -> [w7659]
                tunnel: w7609 -> [w7663]
                tunnel: w7608 -> [w7662]
                tunnel: [w7661] -> w7607
                tunnel: [w7660] -> w7606
                tunnel: [w7657] -> w7591
                tunnel: [w7656] -> w7588
                tunnel: [w7674] -> w7597
                tunnel: w7607 -> [w7675]
                tunnel: w7606 -> [w7676]
                tunnel: [w7673] -> w7595
                tunnel: [w7672] -> w7592
                tunnel: w7591 -> [w7672]
                tunnel: [w7671] -> w7589
                tunnel: w7588 -> [w7671]
                tunnel: w7597 -> [w7684]
                tunnel: [w7684] -> w7596
                tunnel: w7595 -> [w7683]
                tunnel: [w7683] -> w7594
                tunnel: [w7680] -> w7593
                tunnel: w7592 -> [w7682]
                tunnel: [w7679] -> w7590
                tunnel: w7589 -> [w7681]
                tunnel: w7596 -> [w7691]
                tunnel: [w7692] -> w7586
                tunnel: w7594 -> [w7690]
                tunnel: w7593 -> [w7689]
                tunnel: w7590 -> [w7688]
                tunnel: [w7687] -> w7585
                tunnel: [w7686] -> w7584
                tunnel: [w7685] -> w7583
                tunnel: [w7695] -> w7587
                tunnel: w7586 -> [w7695]
                tunnel: w7585 -> [_]
                tunnel: w7584 -> [_]
                tunnel: w7583 -> [_]
                tunnel: w7587 -> [w7702]
                frame #0 {
                  n2269 = call "PID Distance.vi"("Distance"=20.0, "Angle"=0.0, "RightEncoder"=w7624, "LeftEncoder"=w7625, "GyroDevRef"=w7626, "RobotDriveDevRef"=w7627) -> ("RightEncoder 2"=w7620:T11, "LeftEncoder 2"=w7621:T11, "GyroDevRef 2"=w7622:T8, "RobotDriveDevRef 2"=w7623:T1)  [unwired: 2 in]
                }
                frame #1 {
                  n2270 = call "PID Distance.vi"("Distance"=220.0, "Angle"=0.0, "RightEncoder"=w7634, "LeftEncoder"=w7635, "GyroDevRef"=w7637, "RobotDriveDevRef"=w7636) -> ("RightEncoder 2"=w7630:T11, "LeftEncoder 2"=w7631:T11, "GyroDevRef 2"=w7633:T8, "RobotDriveDevRef 2"=w7632:T1)  [unwired: 2 in]
                  n2271 = global write "Robot Global Data.vi" "Raise_Mast"(TRUE ("Current State")) -> ()
                }
                frame #2 {
                  n2272 = call "PID turning.vi"("Angle"=-90.0, "GyroDevRef"=w7643, "RobotDriveDevRef"=w7644) -> ("GyroDevRef 2"=w7642:T8, "RobotDriveDevRef 2"=w7641:T1)  [unwired: 7 in]
                }
                frame #3 {
                  n2273 = call <vilib>:"WPI_EncoderReset.vi"("EncoderDevRef"=w7653) -> ("EncoderDevRef"=w7651:T11)  [unwired: 9 in, 1 out]
                  n2274 = Wait (ms)(milliseconds to wait=u32 10) -> ()  [unwired: 1 out]
                  n2275 = call <vilib>:"WPI_EncoderReset.vi"("EncoderDevRef"=w7654) -> ("EncoderDevRef"=w7652:T11)  [unwired: 9 in, 1 out]
                }
                frame #4 {
                  n2276 = global read "Robot Global Data.vi" "Axes"() -> (w7667:dbl[])
                  n2277 = call "PID Distance.vi"("Distance"=160.0, "Angle"=-90.0, "RightEncoder"=w7658, "LeftEncoder"=w7659, "GyroDevRef"=w7663, "RobotDriveDevRef"=w7662) -> ("RightEncoder 2"=w7656:T11, "LeftEncoder 2"=w7657:T11, "GyroDevRef 2"=w7660:T8, "RobotDriveDevRef 2"=w7661:T1)  [unwired: 2 in]
                  n2278 = global write "Robot Global Data.vi" "Lift_Position"(2.0) -> ()
                  n2279 = Array To Cluster(array=w7667) -> (cluster=w7668:T15)
                  n2280 = Bundle By Name(cluster=w7668, "Axes[1]"=-1.0) -> (w7665:T15)
                  n2281 = Cluster To Array(cluster=w7665) -> (array=w7666:dbl[])
                  n2282 = global write "Robot Global Data.vi" "Axes"(w7666) -> ()
                }
                frame #5 {
                  n2283 = call "PID turning.vi"("Angle"=-180.0, "GyroDevRef"=w7676, "RobotDriveDevRef"=w7675) -> ("GyroDevRef 2"=w7673:T8, "RobotDriveDevRef 2"=w7674:T1)  [unwired: 7 in]
                }
                frame #6 {
                  n2284 = call <vilib>:"WPI_EncoderReset.vi"("EncoderDevRef"=w7682) -> ("EncoderDevRef"=w7680:T11)  [unwired: 9 in, 1 out]
                  n2285 = Wait (ms)(milliseconds to wait=u32 10) -> ()  [unwired: 1 out]
                  n2286 = call <vilib>:"WPI_EncoderReset.vi"("EncoderDevRef"=w7681) -> ("EncoderDevRef"=w7679:T11)  [unwired: 9 in, 1 out]
                }
                frame #7 {
                  n2287 = call "PID Distance.vi"("Distance"=20.0, "Angle"=-180.0, "RightEncoder"=w7688, "LeftEncoder"=w7689, "GyroDevRef"=w7690, "RobotDriveDevRef"=w7691) -> ("RightEncoder 2"=w7685:T11, "LeftEncoder 2"=w7686:T11, "GyroDevRef 2"=w7687:T8, "RobotDriveDevRef 2"=w7692:T1)  [unwired: 2 in]
                }
                frame #8 {
                  n2288 = global read "Robot Global Data.vi" "Axes"() -> (w7697:dbl[])
                  n2289 = Array To Cluster(array=w7697) -> (cluster=w7696:T15)
                  n2290 = Bundle By Name(cluster=w7696, "Axes[1]"=1.0) -> (w7699:T15)
                  n2291 = Cluster To Array(cluster=w7699) -> (array=w7698:dbl[])
                  n2292 = global write "Robot Global Data.vi" "Axes"(w7698) -> ()
                }
                frame #9 {
                  w7709 = 0.0 ("Left axis value")
                  n2293 = global read "Robot Global Data.vi" "Axes"() -> (w7705:dbl[])
                  n2294 = call <vilib>:"WPI_RobotDriveTankDrive.vi"("Right axis value"=w7709, "Left axis value"=w7709, "RobotDriveDevRef"=w7702) -> ()  [unwired: 6 in, 3 out]
                  n2295 = global write "Robot Global Data.vi" "Lift_Position"(3.0) -> ()
                  n2296 = Wait (ms)(milliseconds to wait=u32 10) -> ()  [unwired: 1 out]
                  n2297 = Array To Cluster(array=w7705) -> (cluster=w7704:T15)
                  n2298 = Bundle By Name(cluster=w7704, "Axes[1]"=1.0) -> (w7707:T15)
                  n2299 = Cluster To Array(cluster=w7707) -> (array=w7706:dbl[])
                  n2300 = global write "Robot Global Data.vi" "Axes"(w7706) -> ()
                }
                frame #10 {
                  n2301 = global write "Robot Global Data.vi" "Current State"(FALSE ("Current State")) -> ()
                }
              }
            }
            frame Default {
              n2302 = flat-sequence {
                tunnel: w7714 -> [w7720]
                tunnel: w7713 -> [w7719]
                tunnel: w7712 -> [w7717]
                tunnel: [w7718] -> w7715
                tunnel: w7711 -> [w7716]
                tunnel: w7715 -> [w7723]
                frame #0 {
                  n2303 = call "PID Distance.vi"("Distance"=90.0, "Angle"=0.0, "RightEncoder"=w7716, "LeftEncoder"=w7717, "GyroDevRef"=w7719, "RobotDriveDevRef"=w7720) -> ("RobotDriveDevRef 2"=w7718:T1)  [unwired: 2 in, 3 out]
                }
                frame #1 {
                  w7724 = 0.0
                  n2304 = call <vilib>:"WPI_RobotDriveTankDrive.vi"("Right axis value"=w7724, "Left axis value"=w7724, "RobotDriveDevRef"=w7723) -> ()  [unwired: 6 in, 3 out]
                }
              }
            }
          }
        }
      }
    }
    frame "Test Angle" {
      n2305 = flat-sequence {
        tunnel: w7731 -> [w7739]
        tunnel: w7730 -> [w7738]
        tunnel: w7729 -> [w7737]
        tunnel: w7728 -> [w7736]
        tunnel: [w7733] -> w7727
        tunnel: [w7732] -> w7726
        tunnel: w7727 -> [w7742]
        tunnel: w7726 -> [w7741]
        tunnel: w7725 -> [w7740]
        frame #0 {
          w7735 = 0.0 ("Left axis value")
          n2306 = call <vilib>:"WPI_EncoderReset.vi"("EncoderDevRef"=w7737) -> ()  [unwired: 9 in, 2 out]
          n2307 = call <vilib>:"WPI_EncoderReset.vi"("EncoderDevRef"=w7736) -> ()  [unwired: 9 in, 2 out]
          n2308 = Wait (ms)(milliseconds to wait=u32 10) -> ()  [unwired: 1 out]
          n2309 = call <vilib>:"WPI_GyroReset.vi"("GyroDevRef"=w7739) -> ("GyroDevRef"=w7732:T8)  [unwired: 9 in, 1 out]
          n2310 = call <vilib>:"WPI_RobotDriveTankDrive.vi"("Right axis value"=w7735, "Left axis value"=w7735, "RobotDriveDevRef"=w7738) -> ("RobotDriveDevRef"=w7733:T1)  [unwired: 6 in, 2 out]
        }
        frame #1 {
          n2311 = while {
            shift-right: [w7744] -> _
            shift-left: w7741 -> [w7747]
            shift-right: [w7745] -> _
            shift-left: w7742 -> [w7748]
            shift-right: [w7743] -> _
            shift-left: w7740 -> [w7743]
            stop <- FALSE stop-if-true
            n2312 = call "PID turning.vi"("Angle"=w7743, "GyroDevRef"=w7747, "RobotDriveDevRef"=w7748) -> ("GyroDevRef 2"=w7744:T8, "RobotDriveDevRef 2"=w7745:T1)  [unwired: 7 in]
          }
        }
      }
    }
    frame "Test Distance" {
      n2313 = flat-sequence {
        tunnel: [w7766] -> w7758
        tunnel: [w7765] -> w7757
        tunnel: w7756 -> [w7764]
        tunnel: w7755 -> [w7763]
        tunnel: w7754 -> [w7762]
        tunnel: w7753 -> [w7761]
        tunnel: [w7760] -> w7752
        tunnel: [w7759] -> w7751
        tunnel: w7758 -> [w7774]
        tunnel: w7757 -> [w7773]
        tunnel: w7752 -> [w7772]
        tunnel: w7751 -> [w7771]
        tunnel: w7750 -> [w7770]
        tunnel: w7749 -> [w7769]
        frame #0 {
          w7768 = 0.0 ("Left axis value")
          n2314 = call <vilib>:"WPI_EncoderReset.vi"("EncoderDevRef"=w7762) -> ("EncoderDevRef"=w7760:T11)  [unwired: 9 in, 1 out]
          n2315 = call <vilib>:"WPI_EncoderReset.vi"("EncoderDevRef"=w7761) -> ("EncoderDevRef"=w7759:T11)  [unwired: 9 in, 1 out]
          n2316 = Wait (ms)(milliseconds to wait=u32 10) -> ()  [unwired: 1 out]
          n2317 = call <vilib>:"WPI_GyroReset.vi"("GyroDevRef"=w7763) -> ("GyroDevRef"=w7765:T8)  [unwired: 9 in, 1 out]
          n2318 = call <vilib>:"WPI_RobotDriveTankDrive.vi"("Right axis value"=w7768, "Left axis value"=w7768, "RobotDriveDevRef"=w7764) -> ("RobotDriveDevRef"=w7766:T1)  [unwired: 6 in, 2 out]
        }
        frame #1 {
          n2319 = while {
            shift-right: [w7781] -> _
            shift-left: w7773 -> [w7782]
            shift-right: [w7783] -> _
            shift-left: w7774 -> [w7784]
            shift-right: [w7779] -> _
            shift-left: w7772 -> [w7780]
            shift-right: [w7777] -> _
            shift-left: w7771 -> [w7778]
            shift-right: [w7776] -> _
            shift-left: w7770 -> [w7776]
            shift-right: [w7775] -> _
            shift-left: w7769 -> [w7775]
            stop <- FALSE stop-if-true
            n2320 = call "PID Distance.vi"("Distance"=w7775, "Angle"=w7776, "RightEncoder"=w7778, "LeftEncoder"=w7780, "GyroDevRef"=w7782, "RobotDriveDevRef"=w7784) -> ("RightEncoder 2"=w7777:T11, "LeftEncoder 2"=w7779:T11, "GyroDevRef 2"=w7781:T8, "RobotDriveDevRef 2"=w7783:T1)  [unwired: 2 in]
          }
        }
      }
    }
    frame "Test Vision" {
      n2321 = flat-sequence {
        tunnel: [w7803] -> w7794
        tunnel: [w7802] -> w7793
        tunnel: [w7801] -> w7792
        tunnel: [w7800] -> w7791
        tunnel: w7789 -> [w7799]
        tunnel: w7788 -> [w7798]
        tunnel: w7787 -> [w7797]
        tunnel: w7786 -> [w7796]
        tunnel: w7794 -> [w7806]
        tunnel: w7793 -> [_]
        tunnel: w7792 -> [_]
        tunnel: w7791 -> [_]
        tunnel: w7790 -> [_]
        frame #0 {
          w7805 = 0.0 ("Left axis value")
          n2322 = call <vilib>:"WPI_GyroReset.vi"("GyroDevRef"=w7797) -> ("GyroDevRef"=w7802:T8)  [unwired: 9 in, 1 out]
          n2323 = call <vilib>:"WPI_EncoderReset.vi"("EncoderDevRef"=w7798) -> ("EncoderDevRef"=w7801:T11)  [unwired: 9 in, 1 out]
          n2324 = call <vilib>:"WPI_EncoderReset.vi"("EncoderDevRef"=w7799) -> ("EncoderDevRef"=w7800:T11)  [unwired: 9 in, 1 out]
          n2325 = global write "Robot Global Data.vi" "Current State"(FALSE ("Previous State")) -> ()
          n2326 = Wait (ms)(milliseconds to wait=u32 10) -> ()  [unwired: 1 out]
          n2327 = call <vilib>:"WPI_RobotDriveTankDrive.vi"("Right axis value"=w7805, "Left axis value"=w7805, "RobotDriveDevRef"=w7796) -> ("RobotDriveDevRef"=w7803:T1)  [unwired: 6 in, 2 out]
        }
        frame #1 {
          n2328 = while {
            shift-right: [w7808] -> _
            shift-left: w7806 -> [w7809]
            stop <- FALSE stop-if-true
            n2329 = call "PID vision.vi"("RobotDriveDevRef in"=w7809) -> ("RobotDriveDevRef out"=w7808:T1)  [unwired: 9 in, 1 out]
          }
        }
      }
    }
    frame "Test Infrared" {
      n2330 = flat-sequence {
        tunnel: [w7829] -> w7820
        tunnel: [w7828] -> w7819
        tunnel: [w7827] -> w7818
        tunnel: [w7826] -> w7817
        tunnel: w7813 -> [w7825]
        tunnel: w7814 -> [w7824]
        tunnel: w7812 -> [w7823]
        tunnel: w7811 -> [w7822]
        tunnel: w7820 -> [w7838]
        tunnel: w7819 -> [w7837]
        tunnel: w7818 -> [w7833]
        tunnel: w7817 -> [w7832]
        tunnel: w7816 -> [w7835]
        tunnel: w7815 -> [w7836]
        tunnel: w7810 -> [w7834]
        frame #0 {
          w7831 = 0.0 ("Left axis value")
          n2331 = call <vilib>:"WPI_EncoderReset.vi"("EncoderDevRef"=w7824) -> ("EncoderDevRef"=w7827:T11)  [unwired: 9 in, 1 out]
          n2332 = global write "Robot Global Data.vi" "Current State"(FALSE ("Previous State")) -> ()
          n2333 = Wait (ms)(milliseconds to wait=u32 10) -> ()  [unwired: 1 out]
          n2334 = call <vilib>:"WPI_GyroReset.vi"("GyroDevRef"=w7823) -> ("GyroDevRef"=w7828:T8)  [unwired: 9 in, 1 out]
          n2335 = call <vilib>:"WPI_EncoderReset.vi"("EncoderDevRef"=w7825) -> ("EncoderDevRef"=w7826:T11)  [unwired: 9 in, 1 out]
          n2336 = call <vilib>:"WPI_RobotDriveTankDrive.vi"("Right axis value"=w7831, "Left axis value"=w7831, "RobotDriveDevRef"=w7822) -> ("RobotDriveDevRef"=w7829:T1)  [unwired: 6 in, 2 out]
        }
        frame #1 {
          n2337 = while {
            shift-right: [w7849] -> _
            shift-left: w7838 -> [w7850]
            shift-right: [w7847] -> _
            shift-left: w7837 -> [w7848]
            shift-right: [w7845] -> _
            shift-left: w7836 -> [w7846]
            shift-right: [w7844] -> _
            shift-left: w7835 -> [w7844]
            shift-right: [w7841] -> _
            shift-left: w7832 -> [w7842]
            shift-right: [w7840] -> _
            shift-left: w7833 -> [w7843]
            shift-right: [w7839] -> _
            shift-left: w7834 -> [w7839]
            stop <- FALSE stop-if-true
            n2338 = call "PID with Infrared.vi"("RobotDriveDevRef"=w7850, "Angle"=w7844, "Encoder Limit"=w7839, "GyroDevRef"=w7848, "Left Encoder"=w7843, "Right Encoder"=w7842, "DigitalInputDevRef"=w7846) -> ("RobotDriveDevRef 2"=w7849:T1, "GyroDevRef 2"=w7847:T8, "Left Encoder 2"=w7840:T11, "Right Encoder 2"=w7841:T11, "DigitalInputDevRef 2"=w7845:T7)  [unwired: 4 in]
          }
        }
      }
    }
  }
